vi "test-orient.vi"() -> ()   [LabVIEW 2019]
uses:
  <vilib>/Rock Robotics/WPI/ThirdParty/JAS_Junk/TrajLib/TypeDef/ROTATION2D.ctl
  <vilib>/Rock Robotics/WPI/ThirdParty/JAS_Junk/TrajLib/Trajectory_Library.lvlib
panel:
  out "Loop Count":i32
  in  "Starting Orientation":T1 {"SIN" format="%13.4f"; "COS" format="%13.4f"; "VALUE" format="%13.4f"}
  in  "End Orientation Demand DEG":dbl
  in  "Time Fraction":dbl step=0.01
  in  "Init":bool
  in  "Completion Fraction":dbl=0.8
  out "Orientation Demand Deg":dbl
  out "Orientation Demand":T1 {"SIN" format="%13.4f"; "COS" format="%13.4f"; "VALUE" format="%13.4f"}
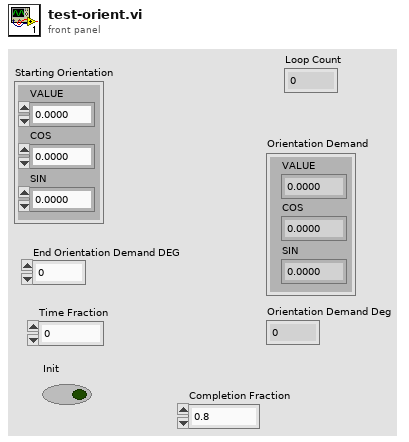
[diagram p1: front panel]
types:
  T1 = typedef "Trajectory_Library.lvlib/ROTATION2D.ctl" = cluster{"VALUE":dbl, "COS":dbl, "SIN":dbl}
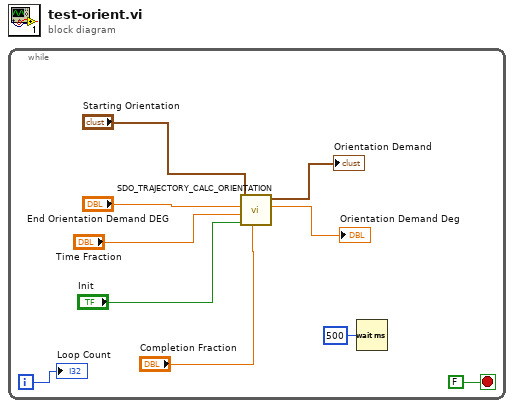
[diagram p0: block diagram]
diagram:
  n1 = while {
    i -> [w1]
    stop <- FALSE stop-if-true
    n2 = call "SDO_TRAJECTORY_CALC_ORIENTATION.vi"("Completion Fraction"="Completion Fraction", "Init"="Init", "Time Fraction"="Time Fraction", "End Orientation Demand DEG"="End Orientation Demand DEG", "Starting Orientation"="Starting Orientation") -> ("Orientation Demand Deg"=→"Orientation Demand Deg":dbl, "Orientation Demand"=→"Orientation Demand":T1)  [unwired: 5 in]
    n3 = Wait (ms)(milliseconds to wait=u32 500) -> ()  [unwired: 1 out]
    "Loop Count" <- w1
  }
